vi "Panel2(SubVI).vi"() -> ()   [LabVIEW 2019]
uses:
  VARIABLES_GLOBAL.vi
panel:
  in  "selección archivo":bool
  in  "stop":bool
  in  "Filename":path=path "test.lvm"
  in  "PH":dbl
  in  "HUMEDAD":dbl
  in  "TEMPERATURA":dbl
  # "INTRODUCCIÓN DE PARÁMETROS"
  # "INTRODUZCA LOS VALORES OBJETIVO PARA EL CONTROL DEL VIVERO CON UN MÁXIMO DE DOS DECIMALES, UNA VEZ COMPLETADO PULSE EL BOTÓN DE STOP."
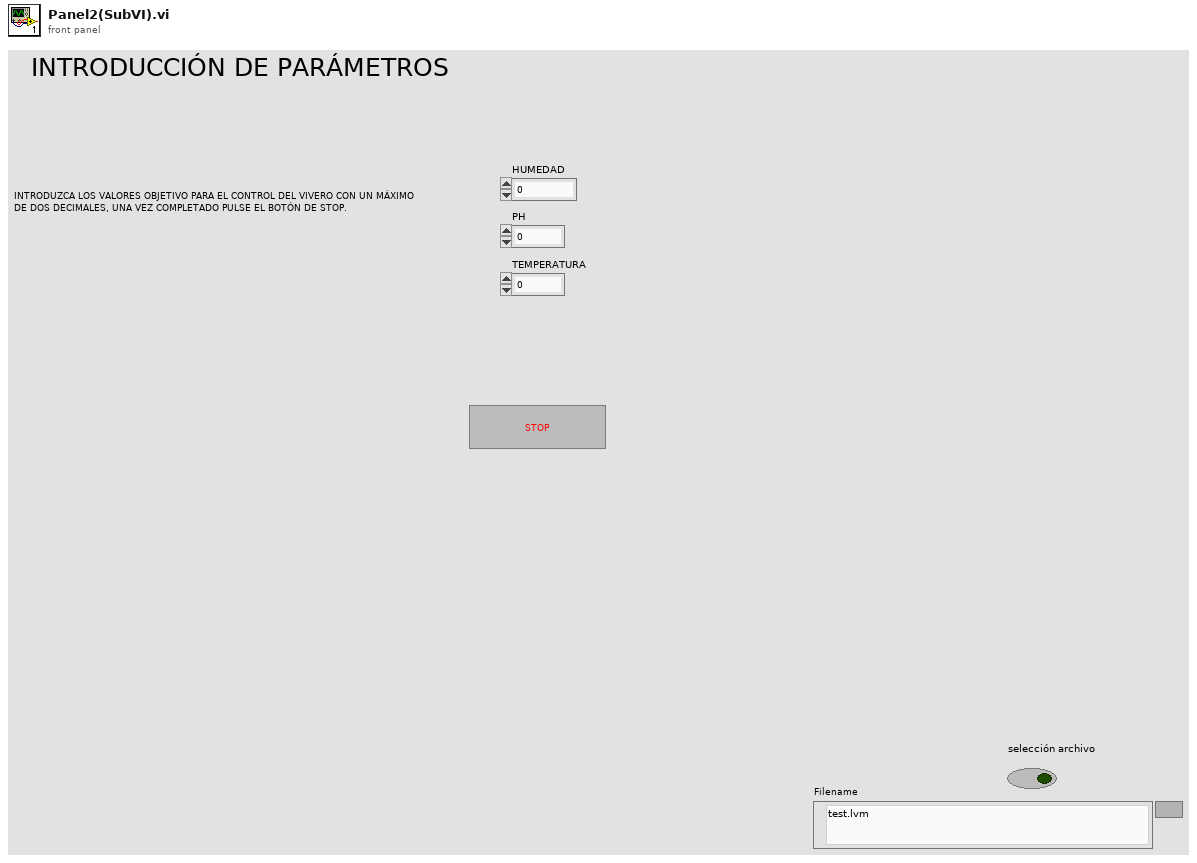
[diagram p1: front panel]
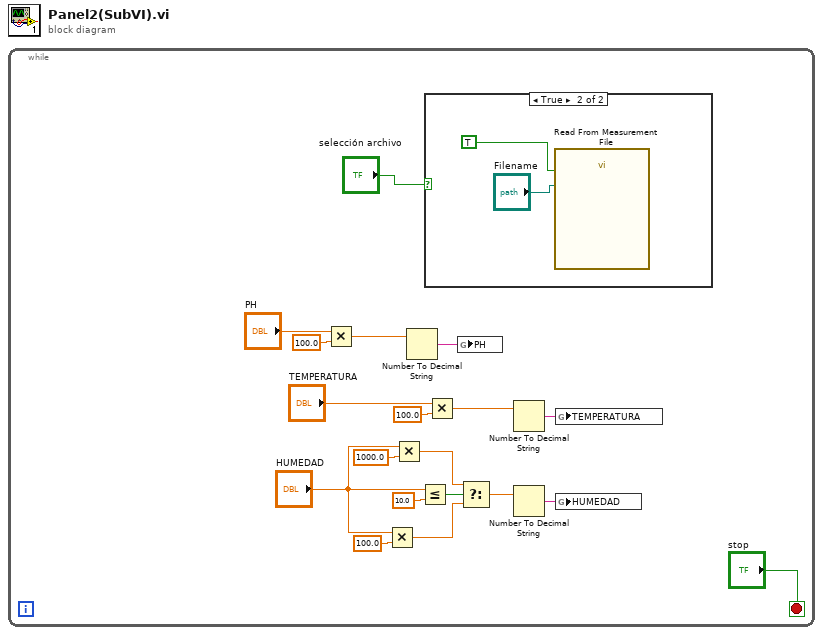
[diagram p0: block diagram]
diagram:
  n1 = while {
    stop <- "stop" stop-if-true
    n2 = Multiply(x="PH", y=100.0) -> (x*y=w3:dbl)
    n3 = Multiply(x="HUMEDAD", y=100.0) -> (x*y=w11:dbl)
    n4 = Multiply(x="HUMEDAD", y=1000.0) -> (x*y=w12:dbl)
    n5 = Number To Decimal String(number=w3) -> (decimal integer string=w2:string)  [unwired: 1 in]
    n6 = Less Or Equal?(x="HUMEDAD", y=10.0) -> (x <= y?=w16:bool)
    n7 = case shown="True" "selección archivo" {
      frame False {
      }
      frame True {
        n8 = call "Read From Measurement File"("Filename"="Filename", "Enable"=TRUE) -> ()  [unwired: 4 in, 6 out]
      }
    }
    n9 = Multiply(x="TEMPERATURA", y=100.0) -> (x*y=w6:dbl)
    n10 = global write "VARIABLES_GLOBAL.vi" "PH"(w2) -> ()
    n11 = Select(t=w12, s=w16, f=w11) -> (s? t:f=w10:dbl)
    n12 = Number To Decimal String(number=w6) -> (decimal integer string=w18:string)  [unwired: 1 in]
    n13 = Number To Decimal String(number=w10) -> (decimal integer string=w9:string)  [unwired: 1 in]
    n14 = global write "VARIABLES_GLOBAL.vi" "TEMPERATURA"(w18) -> ()
    n15 = global write "VARIABLES_GLOBAL.vi" "HUMEDAD"(w9) -> ()
  }
